vi "Size.vi"(8 "error in (no error)":errorcluster, 11 "U32 Array in":refnum<class "U32 Array.lvclass">) -> (0 "error out":errorcluster, 2 "Size":i32, 3 "U32 Array out":refnum<class "U32 Array.lvclass">)   [LabVIEW 2020, in "Data.lvlib" / "U32 Array.lvclass"]
doc: "Return the size of the generic data element."
uses:
  U32 Array.lvclass
  U32 Array.lvclass/U32 Array.ctl
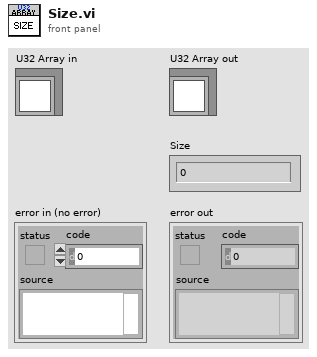
[diagram p1: front panel]
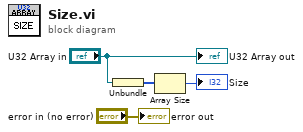
[diagram p0: block diagram]
diagram:
  n1 = Unbundle("U32 Array in") -> (w2:u32[])
  n2 = Array Size(array=w2) -> (size(s)=→"Size":i32)
  "error out" <- "error in (no error)"
  "U32 Array out" <- "U32 Array in"
